vi "FTW-Endpoint-IncomingRequestProxy-Start.vi"(0 "FTW Endpoint":refnum<class "FTW-Endpoint.lvclass">, 11 "error in":errorcluster) -> (4 "FTW Endpoint out":refnum<class "FTW-Endpoint.lvclass">, 6 "Incoming Requests":refnum<event-registration>, 15 "error out":errorcluster)   [LabVIEW 2012, in "FTW-Actor.lvlib" / "FTW-Endpoint.lvclass"]
uses:
  FTW-Endpoint.lvclass
  Message/Request/FTW-Message-IncomingRequest.lvclass
  FTW-Actor.lvlib
panel:
  # "Inputs"
  # "Outputs"
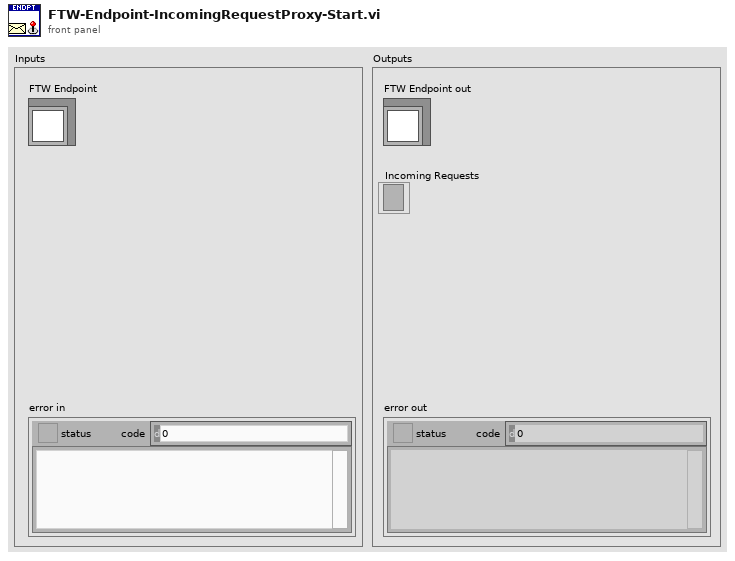
[diagram p1: front panel]
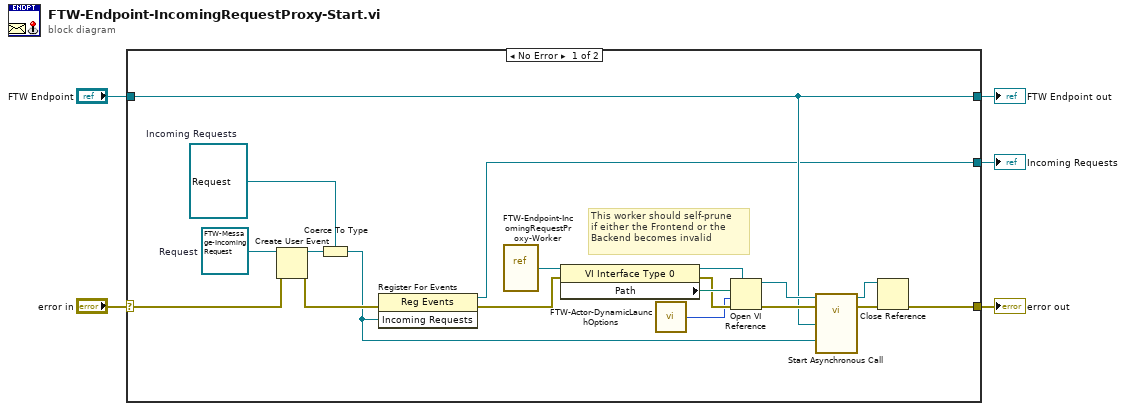
[diagram p0: block diagram]
diagram:
  n1 = case shown="No Error" "error in" {
    selector: "error in" -> [w11 w26]
    tunnel: [w7 w26] -> w5
    tunnel: "FTW Endpoint" -> [w17 w25]
    tunnel: [w17 w25] -> w2
    tunnel: [w6 _] -> w1
    frame No Error {
      w13 = refnum<user-event> refnum  # Incoming Requests
      w14 = refnum<class "FTW-Message-IncomingRequest.lvclass"> refnum  # Request
      # "This worker should self-prune\nif either the Frontend or the\nBackend becomes invalid"
      n2 = Create User Event(user event datatype=w14, error in=w11) -> (user event=w15:refnum<user-event>, error out=w16:errorcluster)
      n3 = Coerce To Type(0:w15, 1:w13) -> (2:w12:refnum<user-event>)
      n4 = register-events(error in=w16, w12) -> (reference out=w6:refnum<event-registration>, error out=w10:errorcluster)  [unwired: 1 in]
      n5 = vi-ref "FTW-Endpoint-IncomingRequestProxy-Worker.vi"() -> (w24:refnum<vi>)
      n6 = property class="VI Interface Type 0"(reference=w24, error in=w10) -> (reference out=w23:refnum<vi>, error out=w20:errorcluster, "Path"=w22:path)
      n7 = call "FTW-Actor-DynamicLaunchOptions.vi"() -> ("Open VI Ref Options"=w19:i32)
      n8 = Open VI Reference(type specifier VI Refnum (for type only)=w23, vi path=w22, options=w19, error in (no error)=w20) -> (vi reference=w18:refnum<vi>, error out=w21:errorcluster)  [unwired: 2 in]
      n9 = call-by-ref "Start Asynchronous Call"(reference=w18, error in=w21, "Backend"=w12, "Frontend Endpoint"=w17) -> (reference out=w9:refnum<vi>, error out=w8:errorcluster)  [unwired: 1 in]
      n10 = Close Reference(reference=w9, error in (no error)=w8) -> (error out=w7:errorcluster)
    }
    frame Error {
    }
  }
  "error out" <- w5
  "FTW Endpoint out" <- w2
  "Incoming Requests" <- w1
